vi "LVClass_ComputePhaseSet ctor from HasoData.vi"(0 "ComputePhaseSet in":refnum<class "ComputePhaseSet.lvclass">, 5 "HasoData.lvclass":refnum<class "HasoData.lvclass">, 11 "error in (no error)":errorcluster) -> (4 "ComputePhaseSet out":refnum<class "ComputePhaseSet.lvclass">, 15 "error out":errorcluster)   [LabVIEW 2020, in "ComputePhaseSet.lvclass"]
doc: "ComputePhaseSet constructor from HasoData. Provide a pointer to a\nComputePhaseSet object adress and a TypePhase value. the TypePhase value\ndepends to the phase recontruction mode of the HasoData.\n\n--------------------------------------------------------------------------------\n\n<B>ComputePhaseSetIn </B> : Constant Pointer to ComputePhaseSet object.\n<B>ComputePhaseSetOut </B> : Constant Pointer to ComputePhaseSet object.\n<B>HasoData </B> : HasoData object.\n<B>TypePhase </B> : TypePhase Polynomial bases enumeration.\n<B>ErrorIn </B> : Error\n<B>ErrorOut </B> : Error\n\n--------------------------------------------------------------------------------"
uses:
  ComputePhaseSet.lvclass
  HasoData.lvclass
  Handle creation.ctl
  ComputePhaseSet.lvclass/ComputePhaseSet.ctl
  LVClass_HasoData Read HasoData - property.vi
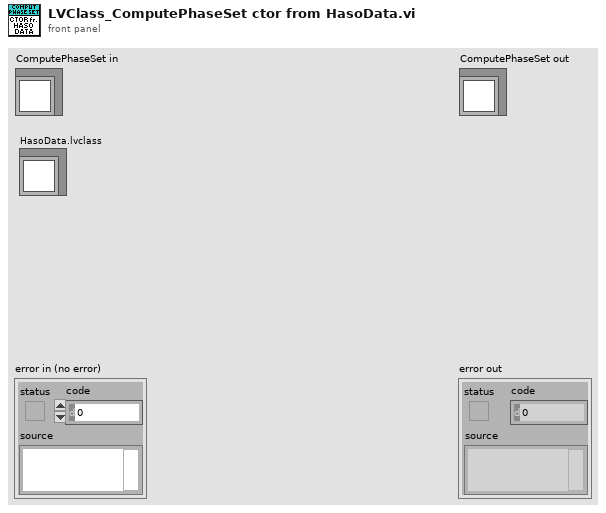
[diagram p1: front panel]
types:
  T1 = typedef "Handle creation.ctl" = enum16{"By ctor", "By write function"}
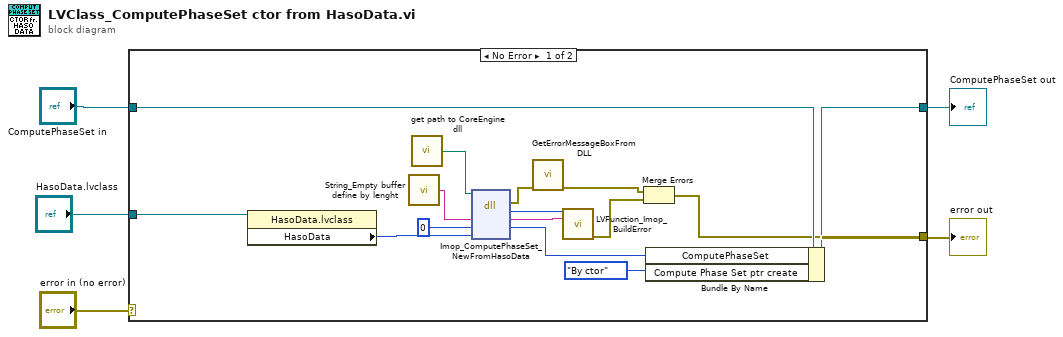
[diagram p0: block diagram]
diagram:
  n1 = case shown="No Error" "error in (no error)" {
    selector: "error in (no error)" -> [_ w22]
    tunnel: [w6 w22] -> w2
    tunnel: [w16 w21] -> w4
    tunnel: "ComputePhaseSet in" -> [w17 w21]
    tunnel: "HasoData.lvclass" -> [w12 _]
    frame No Error {
      n2 = property class="HasoData.lvclass"(reference=w12) -> ("HasoData"=w10:i32)  [unwired: 1 in, 2 out]
      n3 = call "String_Empty buffer define by lenght.vi"() -> ("Empty buffer"=w15:string)  [unwired: 1 in]
      n4 = call "get path to CoreEngine dll.vi"() -> ("path to c_interface_vc100.dll"=w14:path)  [unwired: 12 in, 3 out]
      n5 = dll-call lib="D:/soft/HASO_v3/SVN_trunk/ImOpCoreEngine4_LV2011/DLLs/c_interface_vc100.dll" fn="Imop_ComputePhaseSet_NewFromHasoData"(path in=w14, "message"=w15, "compute phase set"=0 ("objet"), "haso data"=w10) -> (error out=w13:errorcluster, "return type"=w19:i32, "message"=w18:string, "compute phase set"=w9:i32)  [unwired: 3 in, 1 out]
      n6 = call "GetErrorMessageBoxFromDLL.vi"("error IN"=w13) -> ("error OUT"=w8:errorcluster)  [unwired: 10 in]
      n7 = call "LVFunction_Imop_BuildError.vi"("code"=w19, "String to Prepend to source (\"\")"=w18) -> ("error out"=w7:errorcluster)  [unwired: 13 in]
      n8 = Merge Errors(w8, w7) -> (w6:errorcluster)
      n9 = Bundle By Name(cluster=w17, "ComputePhaseSet"=w9, "Compute Phase Set ptr create"=Handle_creation."By ctor" ("Haso ptr create")) -> (w16:refnum<class "ComputePhaseSet.lvclass">)
    }
    frame Error {
    }
  }
  "error out" <- w2
  "ComputePhaseSet out" <- w4
